vi "launchFrontEnd.vi"(8 "error in (no error)":errorcluster, 11 "CamaraSettings in":refnum<class "CamaraSettings.lvclass">) -> (0 "error out":errorcluster, 3 "CamaraSettings out":refnum<class "CamaraSettings.lvclass">)   [LabVIEW 2009, in "Tools.lvlib" / "Settings.lvlib" / "CamaraSettings.lvclass"]
uses:
  CamaraSettings.lvclass
  CamaraSettings.lvclass/CamaraSettings.ctl
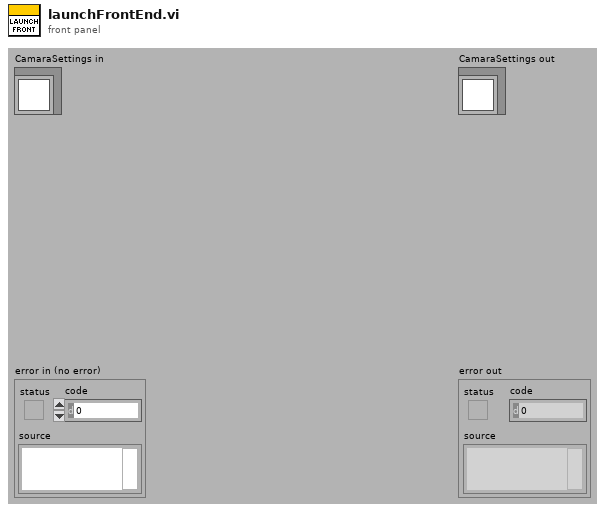
[diagram p1: front panel]
types:
  T1 = enum32{"Invalid", "Standard", "Closed", "Hidden", "Minimized", "Maximized"}
  T2 = enum32{"Bad", "Idle", "Run top level", "Running"}
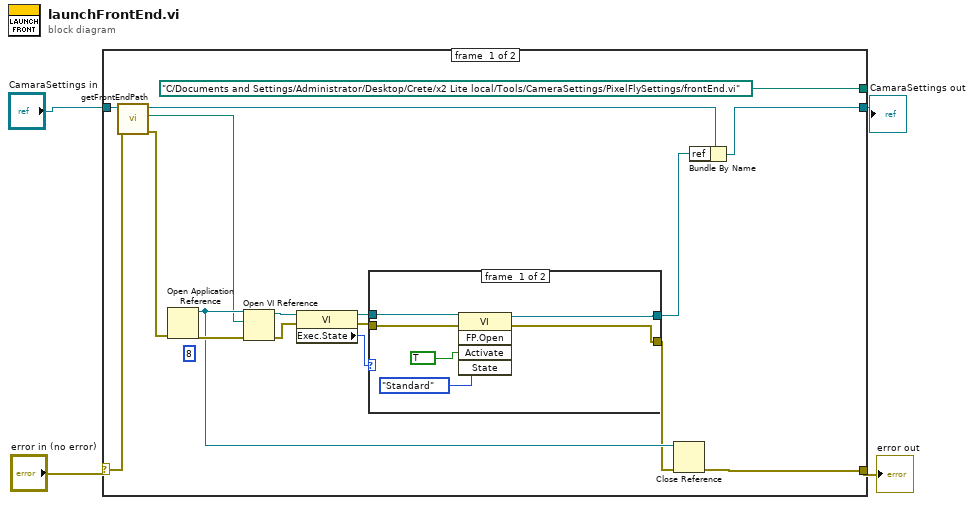
[diagram p0: block diagram]
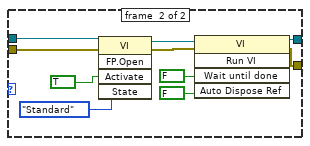
[diagram p2: hidden frame]
diagram:
  n1 = case shown="No Error" "error in (no error)" {
    selector: "error in (no error)" -> [w17 w39]
    tunnel: [w14 w39] -> w3
    tunnel: "CamaraSettings in" -> [w18 w38]
    tunnel: [w12 w38] -> w1
    tunnel: [path "C:/Documents and Settings/Administrator/Desktop/Crete/x2 Lite local/Tools/CameraSettings/PixelFlySettings/frontEnd.vi" _] -> _
    frame #0 {
      (unwired) 8
      n2 = call-dynamic "getFrontEndPath.vi"("error in (no error)"=w17, "CamaraSettings in"=w18) -> ("error out"=w16:errorcluster, "Path"=w15:path, "CamaraSettings out"=w13:refnum<class "CamaraSettings.lvclass">)  [unwired: 7 in]
      n3 = Open Application Reference(8:w16) -> (0:w21:errorcluster, 3:w20:refnum<vi>)  [unwired: 3 in]
      n4 = Open VI Reference(application reference (local)=w20, vi path=w15, error in (no error)=w21) -> (vi reference=w9:refnum<vi>, error out=w10:errorcluster)  [unwired: 3 in]
      n5 = property class="VI"(reference=w9, error in=w10) -> (reference out=w7:refnum<vi>, error out=w8:errorcluster, "Exec.State"=w6:T2)
      n6 = case shown="Default" w6 {
        tunnel: [w22 w35] -> w19
        tunnel: [w23 w31] -> w11
        tunnel: w8 -> [w25 w29]
        tunnel: w7 -> [w24 w28]
        frame #0 {
          n7 = invoke class="VI" method="FP.Open"(reference=w24, error in=w25, "Activate"=TRUE, "State"=T1."Standard") -> (reference out=w23:refnum<vi>, error out=w22:errorcluster)  [unwired: 1 in, 3 out]
        }
        frame #1 {
          n8 = invoke class="VI" method="FP.Open"(reference=w28, error in=w29, "Activate"=TRUE, "State"=T1."Standard") -> (reference out=w30:refnum<vi>, error out=w32:errorcluster)  [unwired: 1 in, 3 out]
          n9 = invoke class="VI" method="Run VI"(reference=w30, error in=w32, "Wait until done"=FALSE, "Auto Dispose Ref"=FALSE) -> (reference out=w31:refnum<vi>, error out=w35:errorcluster)  [unwired: 1 in, 3 out]
        }
      }
      n10 = Close Reference(reference=w20, error in (no error)=w19) -> (error out=w14:errorcluster)
      n11 = Bundle By Name(cluster=w13, "ref"=w11) -> (w12:refnum<class "CamaraSettings.lvclass">)
    }
    frame #1 {
    }
  }
  "error out" <- w3
  "CamaraSettings out" <- w1
